vi "Main.vi"() -> ()   [LabVIEW 2017, in "Client.lvlib"]
uses:
  Client.lvlib
  CommsFrameWork.lvlib
  CommsServer.lvlib
  LabVIEWHTTPClient.lvlib
  ClientErrorHandler.lvlib
  ClientLogger.lvlib
  UI_API.lvlib
panel:
  out "Prio 4":u32(colorbox)
  out "Prio 3":u32(colorbox)
  out "Prio 2":u32(colorbox)
  out "Prio 1":u32(colorbox)
  in  "Filter Preset":T1(ring)
  out "Time to Refresh":dbl(slide) scale=0.0..10.0
  out "Connection Quality":dbl(knob) scale=0.0..10.0
  out "Connected?":bool
  out "Last Update":timestamp
  in  "Refresh":bool
  in  "AE Level":enum16{"AE / ELP", "AE Intern"}(ring)
  in  "AE Groups":i32[](listbox)
  in  "SRs Tab":enum32{"Unassigned", "Assigned", "Debug"}(tab)
  out "Unassigned Sorted SRs":string[][](table)
  out "Assigned Sorted SRs":string[][](table)
  out "INI Content":string
  out "INI Path":path
  in  "Read INI":bool
  out "Last Error Detected":errorcluster
  in  "Text":string="Manual Log Entry"
  in  "Type":string="Event"
  in  "Generate Log Entry":bool
  in  "Injected Error":errorcluster
  in  "Generate Error":bool
  # "Priority 1"
  # "Priority 3"
  # "Priority 2"
  # "Priority 4"
  # "Manual Controls"
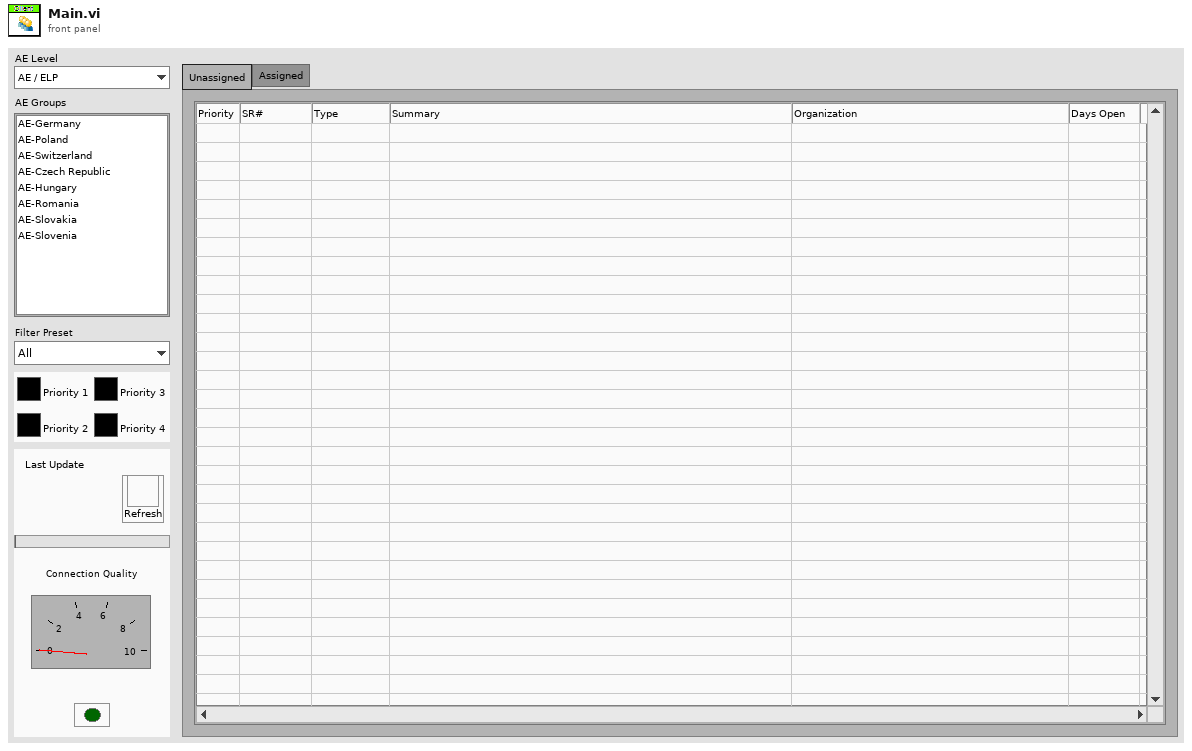
[diagram p1: front panel]
types:
  T1 = enum16{"All", "Eastern Europe", "DACH", "Custom"}
  T2 = cluster{"ErrorEventReg":refnum<event-registration>, "ErrorEvent":refnum<user-event>, "Queues":cluster{"MHLClient":refnum<queue>, "ErrorHandler":refnum<queue>, "EventHandler":refnum<queue>, "ConnectionHandler":refnum<queue>, "UIHandler":refnum<queue>, "Logger":refnum<queue>}}
  T3 = typedef "LVPoint32TypeDef.ctl" = cluster{"Horizontal":i32, "Vertical":i32}
  T4 = cluster{"Assigned SRs":refnum<vi>, "Unassigned SRs":refnum<vi>, "AE Level":refnum<vi>, "AE Groups":refnum<vi>}
  T5 = cluster{"SR Number":i64, "AE Group":enum32{"NaN", "AE-Germany", "AE-Poland", "AE-Switzerland", "AE-Czech Republic", "AE-Hungary", "AE-Romania", "AE-Slovakia", "AE-Slovenia"}, "SR Owner":string, "Summary":string, "SR Status":enum32{"NaN", "Caller Abandoned", "Created in Error", "Declined to Purchase Support", "Expired", "Forum Resolved AE", "Forum Resolved Customer", "IN WORK", "IN WORK Collab with AES", "IN WORK Collab with PSE", "IN WORK Collab with SE", "IN WORK Escalation", "IN WORK Customer Added Note", "Open", "Potentially Resolved", "POC Resolved", "Resolved", "RMA Waiting on Customer", "RMA Open", "RMA In Progress", "RMA Closed - DOA", "RMA Closed", "RMA Approved for Return", "Project Complete", "Presumed Resolved", "IN WORK Wait on Customer"}, "Days Open":dbl, "Prio":enum16{"Prio 1", "Prio 2", "Prio 3", "Prio 4"}, "SR Type":enum32{"NaN", "ATE Core Configurations (BYOATE)", "Activation", "BioBench", "CAN", "CM C Series", "Calibration", "Consulting Services", "CounterTimer", "DAQExpress", "DASYLab", "DIAdem", "DMM", "DSA HW", "Digital_IO", "FIRST (NIC Only)", "FieldBus", "FieldPoint", "Functional Savety", "GATI", "GPIB", "HMI and Industrial PCs", "HiQ", "HighSpeedDigital_IO", "IMAQ", "IOTech Vibration", "Industrial Communications", "InsightCM", "LV", "LV CD&Sim", "LV Comms", "LV Controls Add-Ons", "LV Embedded", "LV MathScript RT", "LV NXG", "LV NXT", "LVDSC", "LVFPGA", "LVPDA and LV Touch Panel", "LVRT", "LabWindows_CVI", "Lookout", "MATRIXx", "MStudioDotNet", "MStudioVisualBasic", "MStudioVisualC", "Measure (Legacy)", "Motion", "MultifunctionDAQ", "Multimedia Test HW/SW", "Multisim (EWB)", "NI Update Service", "OPC Servers", "Optical (OSI)", "PXI Controllers, Chassis, MXI", "PXI Timing and Sync", "Power Supplies and SMUs", "Powertrain Controls", "RAID", "RF", "RF Software", "RIO", "SC Express", "SCC", "SCXI", "SPEEDY-33 (Hyperception)", "STS", "ScopeDigitizers", "Serial", "Signal Sources", "SignalCondOther", "SignalExpress", "Software Defined Intruments", "Sound and Vibration SW", "Switch Executive", "Switches", "TestStand", "USRP", "Ultiboard (EWB)", "VBench", "VI Logger", "VXI_MXI", "VeriStand", "VisionSW", "VolumeLicenseMgr", "WSN", "Web UI Builder", "myRIO"}, "Service Level":string, "Last Updated":timestamp, "First Name":string, "Last Name":string, "Organisation Name":string, "Creation Date":timestamp, "Needs Merging?":bool, "English Flag?":bool}[]
  T6 = cluster{"Connection Quality":dbl, "Last Update":timestamp}
  T7 = enum16{"SR Number", "AE Group", "SR Owner", "Summary", "SR Status", "Days Open", "Prio", "SR Type", "Service Level", "Last Updated", "First Name", "Last Name", "Organisation Name", "Creation Date", "Needs Merging?", "English Flag?"}[]
  T8 = cluster{"Connection Data":cluster{"IP":string, "Port":string, "ClientName":string}}
  T9 = cluster{"SR#":dbl, "Group":string, "Owner":string, "Problem Summary":string, "Last Updated":timestamp, "Customer First Name":string, "Customer Last Name":string, "Company":string, "Created On":timestamp, "SR Type":string, "Status":string, "Service Level":string, "Channel":string, "Days Open":dbl}[]
  T10 = cluster{"IP":string, "Port":string, "ClientName":string}
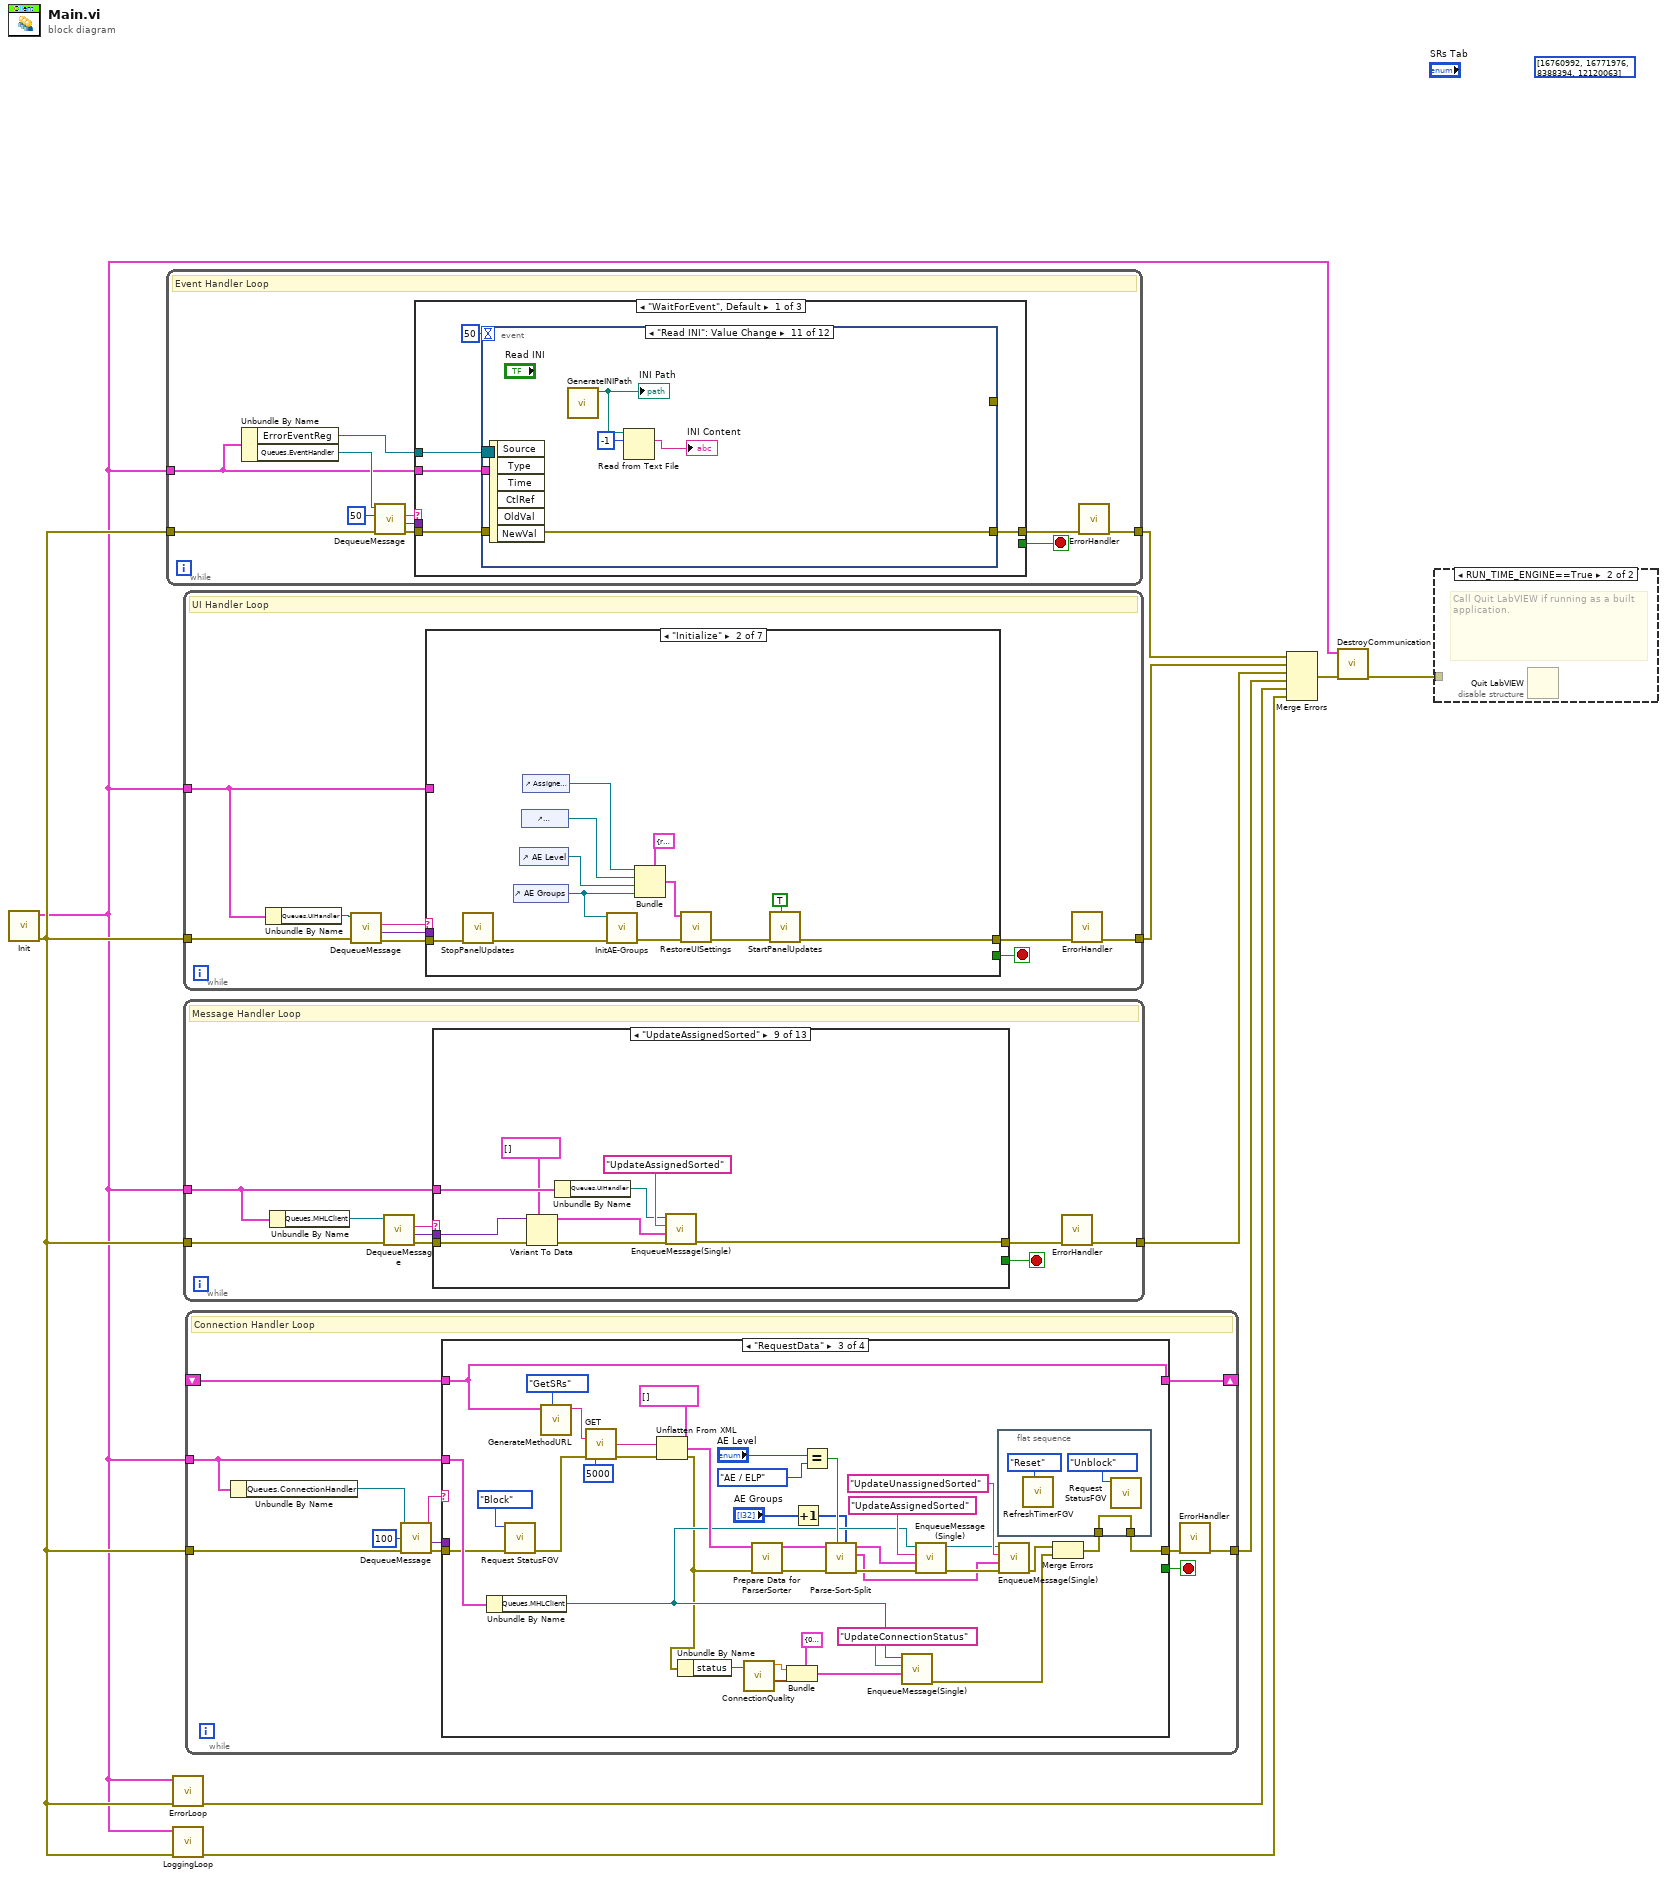
[diagram p0: block diagram]
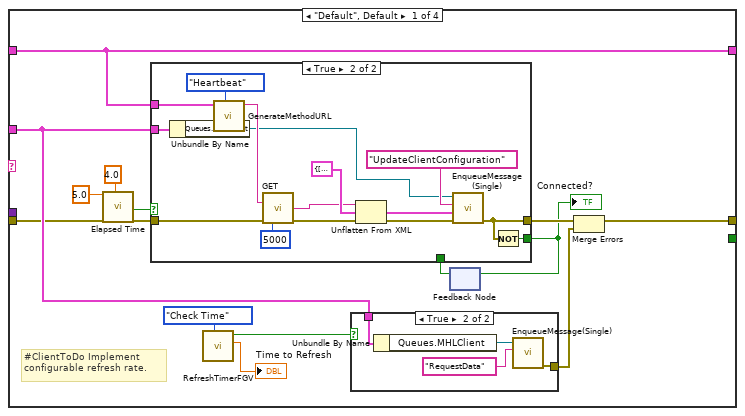
[diagram p2: hidden frame]
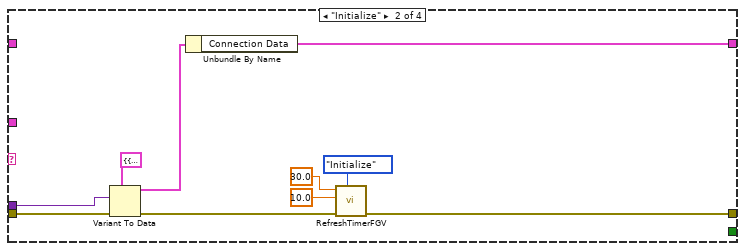
[diagram p5: hidden frame]
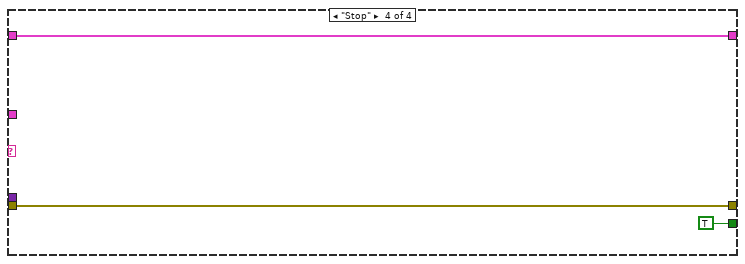
[diagram p6: hidden frame]
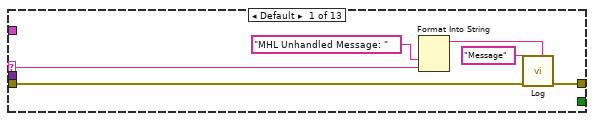
[diagram p7: hidden frame]
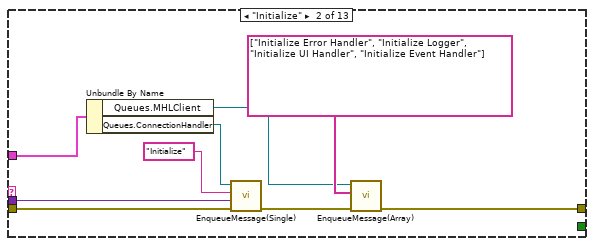
[diagram p8: hidden frame]
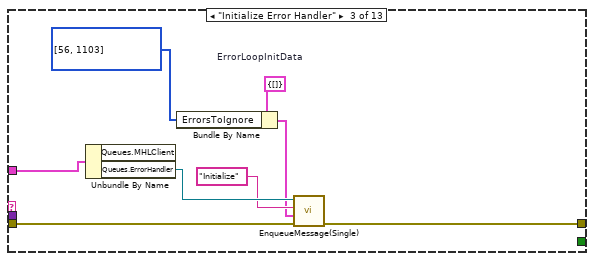
[diagram p9: hidden frame]
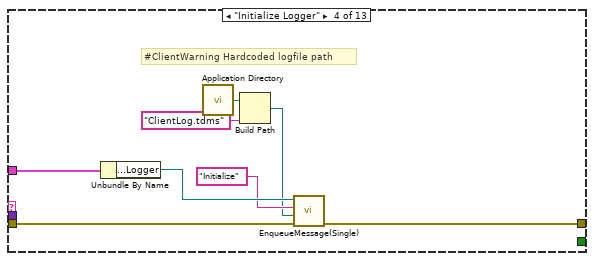
[diagram p10: hidden frame]
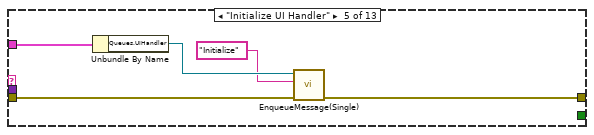
[diagram p11: hidden frame]
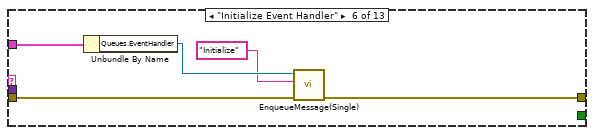
[diagram p12: hidden frame]
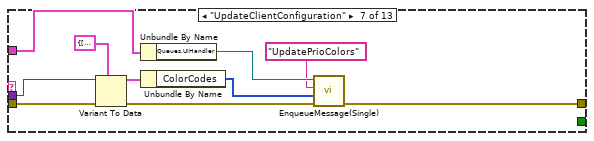
[diagram p13: hidden frame]
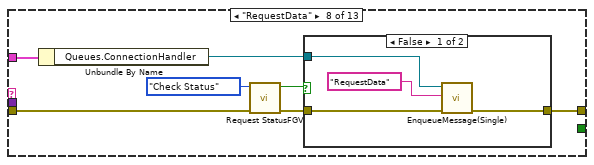
[diagram p14: hidden frame]
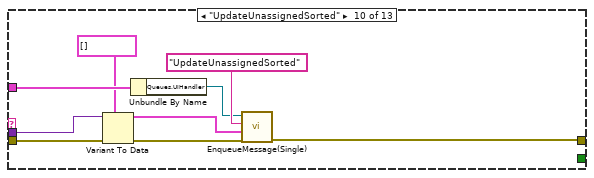
[diagram p16: hidden frame]
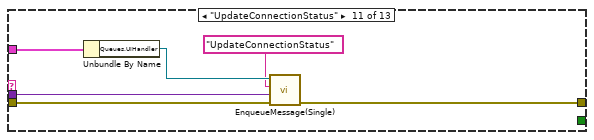
[diagram p17: hidden frame]
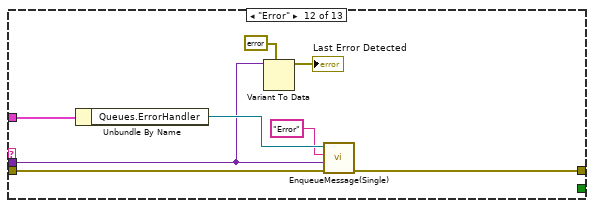
[diagram p18: hidden frame]
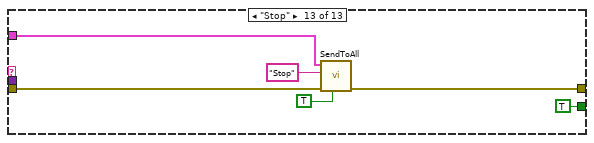
[diagram p19: hidden frame]
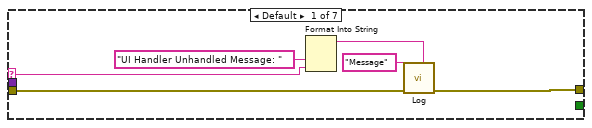
[diagram p20: hidden frame]
diagram:
  (unwired) u32[] [16760992, 16771976, 8388394, 12120063] ("Array")
  n1 = call "Init.vi"() -> ("Error Out"=w4:errorcluster, "Message Queues"=w3:T2)  [unwired: 10 in]
  n2 = while {
    tunnel: w3 -> [w13]
    tunnel: w4 -> [w20]
    tunnel: [w14] -> w9
    stop <- w16 stop-if-true
    # "Event Handler Loop"
    n3 = Unbundle By Name(w13) -> ("ErrorEventReg"=w12:refnum<event-registration>, "Queues.EventHandler"=w21:refnum<queue>)
    n4 = call "DequeueMessage.vi"("error in (no error)"=w20, "timeout ms (-1)"=50, "Message Queue"=w21) -> ("error out"=w18:errorcluster, "Message Data"=w17:variant, "Message"=w19:string)  [unwired: 4 in, 2 out]
    n5 = case shown="\"WaitForEvent\", Default" w19 {
      tunnel: w18 -> [w26 w144 w147]
      tunnel: [w23 w143 w147] -> w15
      tunnel: w17 -> [_ _ _]
      tunnel: [_ _ TRUE] -> w16
      tunnel: w13 -> [w25 w142 _]
      tunnel: w12 -> [w22 _ _]
      frame "WaitForEvent", Default {
        n6 = event shown="[10] \"Read INI\": Value Change" {
          selector: w22 -> [_ _ _ _ _ _ _ _ _ _ _ _]
          dyn-events: _ -> [_ _ _ _ _ _ _ _ _ _ _ _]
          timeout: 50 -> [_ _ _ _ _ _ _ _ _ _ _ _]
          tunnel: w26 -> [w29 w35 w48 w60 w62 w69 w73 w81 w98 w110 w125 w127]
          tunnel: w25 -> [w31 w37 w56 _ _ w68 w75 _ w101 _ _ _]
          tunnel: [w30 w33 w49 w60 w61 w65 w72 w80 w99 w109 w125 w126] -> w23
          tunnel: [_ _ _ _ _ _ w70 _ _ _ _ _] -> _
          event Timeout {
            n7 = event-data() -> ()  [unwired: 1 in, 3 out]
            n8 = Unbundle By Name(w31) -> ("Queues.EventHandler"=w27:refnum<queue>)
            n9 = call "EnqueueMessage(Single).vi"("error in (no error)"=w29, "Message"="WaitForEvent", "Message Queue"=w27) -> ("error out"=w30:errorcluster)  [unwired: 7 in, 1 out]
          }
          event "Filter Preset": Value Change {
            # "#ClientToDo Replace hardwired values with configuration data."
            n10 = event-data() -> ("NewVal"=w38:T1)  [unwired: 1 in]
            n11 = case shown="\"Eastern Europe\"" w38 {
              tunnel: w35 -> [w39 w41 w43 w45]
              tunnel: [w39 w41 w43 w45] -> w34
              frame "All", Default {
                n12 = property on="AE Groups" class="LstBox (strict)"("Value"=i32[] [0, 1, 2, 3, 4, 5, 6, 7] ("Value (Signaling)")) -> ()  [unwired: 2 in, 2 out]
              }
              frame "Eastern Europe" {
                n13 = property on="AE Groups" class="LstBox (strict)"("Value"=i32[] [1, 3, 4, 5, 6, 7] ("Value (Signaling)")) -> ()  [unwired: 2 in, 2 out]
              }
              frame "DACH" {
                n14 = property on="AE Groups" class="LstBox (strict)"("Value"=i32[] [0, 2] ("Value (Signaling)")) -> ()  [unwired: 2 in, 2 out]
              }
              frame "Custom" {
              }
            }
            n15 = Unbundle By Name(w37) -> ("Queues.MHLClient"=w36:refnum<queue>)
            n16 = call "EnqueueMessage(Single).vi"("error in (no error)"=w34, "Message"="RequestData", "Message Queue"=w36) -> ("error out"=w33:errorcluster)  [unwired: 7 in, 1 out]
          }
          event "AE Level", "AE Groups": Value Change {
            n17 = event-data() -> ("CtlRef"=w54:refnum<vi>)  [unwired: 1 in]
            n18 = call "StopPanelUpdates.vi"("Error In"=w48) -> ("Error Out"=w47:errorcluster)  [unwired: 10 in]
            n19 = property class="Ctl"(reference=w54) -> ("Label.Text"=w53:string)  [unwired: 1 in, 2 out]
            n20 = Unbundle By Name(w56) -> ("Queues.MHLClient"=w57:refnum<queue>)
            n21 = case shown="\"AE Groups\"" w53 {
              frame "False", Default {
              }
              frame "AE Groups" {
                n22 = local write "Filter Preset"(T1."Custom" ("Filter Preset")) -> ()
              }
            }
            n23 = call "EnqueueMessage(Single).vi"("error in (no error)"=w47, "Message"="RequestData", "Message Queue"=w57) -> ("error out"=w46:errorcluster)  [unwired: 7 in, 1 out]
            n24 = control-ref of="Unassigned Sorted SRs"() -> (w52:refnum<vi>)
            n25 = control-ref of="Assigned Sorted SRs"() -> (w51:refnum<vi>)
            n26 = Build Array(w52, w51) -> (w50:refnum<vi>[])
            n27 = call "ResetTablesToTopPosition.vi"("Error In"=w46, "Table Refnum Array"=w50) -> ("Error Out"=w49:errorcluster)  [unwired: 9 in]
          }
          event "Generate Error": Value Change {
            # "#ClientWarning Debug Feature"
            n28 = event-data() -> ()  [unwired: 1 in, 6 out]
            n29 = call "ErrorHandler.vi"("error in (no error)"="Injected Error") -> ()  [unwired: 10 in, 1 out]
          }
          event "Generate Log Entry": Value Change {
            # "#ClientWarning Debug Feature"
            n30 = event-data() -> ()  [unwired: 1 in, 6 out]
            n31 = call "Log.vi"("LogMessage"="Text", "Type"="Type", "Error In"=w62) -> ("Error Out"=w61:errorcluster)  [unwired: 8 in]
          }
          event "Refresh": Value Change {
            n32 = event-data() -> ()  [unwired: 1 in, 1 out]
            n33 = Unbundle By Name(w68) -> ("Queues.MHLClient"=w67:refnum<queue>)
            n34 = call "EnqueueMessage(Single).vi"("error in (no error)"=w69, "Message"="RequestData", "Message Queue"=w67) -> ("error out"=w65:errorcluster)  [unwired: 7 in, 1 out]
          }
          event User Event {
            n35 = event-data() -> ("status"=w78:bool, "code"=w77:i32, "source"=w76:string)  [unwired: 1 in]
            n36 = Unbundle By Name(w75) -> ("Queues.MHLClient"=w74:refnum<queue>)
            n37 = Bundle(cluster=errorcluster {"status"=FALSE, "code"=0, "source"=""} ("error constant"), "status"=w78, "code"=w77, "source"=w76) -> (w70:errorcluster)
            n38 = call "EnqueueMessage(Single).vi"("error in (no error)"=w73, "Message"="Stop", "Message Queue"=w74) -> ("error out"=w72:errorcluster)  [unwired: 7 in, 1 out]
          }
          event "Unassigned Sorted SRs": Shortcut Menu Selection (User) {
            # "#ClientToDo Adapt SR# finding to configurable columns"
            n39 = event-data() -> ("ItemTag"=w82:string, "CtlRef"=w84:refnum<vi>, "Coords"=w83:T3)  [unwired: 1 in]
            n40 = case shown="\"Copy SR#\", Default" w82 {
              tunnel: w84 -> [w90 w95]
              tunnel: w83 -> [w89 w93]
              tunnel: [w85 w92] -> w80
              tunnel: w81 -> [w86 w91]
              frame "Open Screenpop" {
                # "#ClientToDo URL from config data."
                n41 = call "Open Screenpop.vi"("Screenpop URL Prefix"="http://force.natinst.com:8000/pls/ebiz/niae_screenpop.main?p_incident_number=", "SR# Cloumn Header"="SR#" ("SR Cloumn Header"), "Error In"=w86, "Coordinates"=w89, "Table Reference"=w90) -> ("Error Out"=w85:errorcluster)  [unwired: 6 in]
              }
              frame "Copy SR#", Default {
                n42 = call "Copy SR Num to Clipboard.vi"("SR Cloumn Header"="SR#", "Error In"=w91, "Coordinates"=w93, "Table Reference"=w95) -> ("Error Out"=w92:errorcluster)  [unwired: 7 in]
              }
            }
          }
          event Panel Close? {
            n43 = event-data() -> ()  [unwired: 1 in, 1 out]
            n44 = Unbundle By Name(w101) -> ("Queues.MHLClient"=w100:refnum<queue>)
            n45 = call "QuitDialog.vi"("Error In"=w98) -> ("Error Out"=w97:errorcluster, "OK Clicked?"=w96:bool)  [unwired: 9 in]
            n46 = case shown="True" w96 {
              tunnel: w100 -> [_ w108]
              tunnel: [w103 w107] -> w99
              tunnel: w97 -> [w103 w106]
              frame False {
              }
              frame True {
                n47 = call "EnqueueMessage(Single).vi"("Priority Message? (F)"=TRUE, "error in (no error)"=w106, "Message"="Stop", "Message Queue"=w108) -> ("error out"=w107:errorcluster)  [unwired: 6 in, 1 out]
              }
            }
            n48 = event-data("Discard?"=TRUE) -> ()  [unwired: 1 in, 1 out]
          }
          event Key Down? {
            # "#ClientWarning Debug Feature"
            n49 = event-data() -> ("ScanCode"=w115:i16, "PlatMods.Ctrl"=w113:bool, "PlatMods.Shift"=w112:bool)  [unwired: 1 in]
            n50 = Equal?(x=i16 32 ("ScanCode"), y=w115) -> (x = y?=w114:bool)
            n51 = Compound Arithmetic op=AND(w114, w113, w112) -> (w111:bool)
            n52 = case shown="True" w111 {
              tunnel: w110 -> [w117 w121]
              tunnel: [w117 w120] -> w109
              frame False {
              }
              frame True {
                n53 = control-ref of="SRs Tab"() -> (w119:refnum<vi>)
                n54 = call "ToggleTab.vi"("Error In"=w121, "Tab Index"=2, "TabCtl Refnum"=w119) -> ("Error Out"=w120:errorcluster)  [unwired: 8 in]
              }
            }
            n55 = event-data() -> ()  [unwired: 2 in, 1 out]
          }
          event "Read INI": Value Change {
            n56 = event-data() -> ()  [unwired: 1 in, 6 out]
            n57 = call "GenerateINIPath.vi"() -> ("INI Path"=w124:path)  [unwired: 11 in]
            "INI Path" <- w124
            n58 = Read from Text File(file (use dialog)=w124, count=-1) -> (text=→"INI Content":string)  [unwired: 2 in, 3 out]
          }
          event "Assigned Sorted SRs": Shortcut Menu Selection (User) {
            # "#ClientToDo Adapt SR# finding to configurable columns"
            n59 = event-data() -> ("ItemTag"=w130:string, "CtlRef"=w129:refnum<vi>, "Coords"=w128:T3)  [unwired: 1 in]
            n60 = case shown="\"Open Screenpop\"" w130 {
              tunnel: w129 -> [w136 w141]
              tunnel: w128 -> [w135 w139]
              tunnel: w127 -> [w132 w138]
              tunnel: [w131 w137] -> w126
              frame "Open Screenpop" {
                # "#ClientToDo URL from config data."
                n61 = call "Open Screenpop.vi"("Screenpop URL Prefix"="http://force.natinst.com:8000/pls/ebiz/niae_screenpop.main?p_incident_number=", "SR# Cloumn Header"="SR#" ("SR Cloumn Header"), "Error In"=w132, "Coordinates"=w135, "Table Reference"=w136) -> ("Error Out"=w131:errorcluster)  [unwired: 6 in]
              }
              frame "Copy SR#", Default {
                n62 = call "Copy SR Num to Clipboard.vi"("SR Cloumn Header"="SR#", "Error In"=w138, "Coordinates"=w139, "Table Reference"=w141) -> ("Error Out"=w137:errorcluster)  [unwired: 7 in]
              }
            }
          }
        }
      }
      frame "Initialize" {
        n63 = Unbundle By Name(w142) -> ("Queues.EventHandler"=w146:refnum<queue>)
        n64 = call "EnqueueMessage(Single).vi"("error in (no error)"=w144, "Message"="WaitForEvent", "Message Queue"=w146) -> ("error out"=w143:errorcluster)  [unwired: 7 in, 1 out]
      }
      frame "Stop" {
      }
    }
    n65 = call "ErrorHandler.vi"("error in (no error)"=w15) -> ("error out"=w14:errorcluster)  [unwired: 10 in]
  }
  n66 = call "ErrorLoop.vi"("Error In"=w4, "Message Queues"=w3) -> ("Error Out"=w5:errorcluster)  [unwired: 9 in]
  n67 = call "LoggingLoop.vi"("Error In"=w4, "Communication References"=w3) -> ("Error Out"=w2:errorcluster)  [unwired: 9 in]
  n68 = while {
    tunnel: w3 -> [w151]
    tunnel: w4 -> [w156]
    tunnel: [w149] -> w8
    stop <- w152 stop-if-true
    # "UI Handler Loop"
    n69 = Unbundle By Name(w151) -> ("Queues.UIHandler"=w157:refnum<queue>)
    n70 = call "DequeueMessage.vi"("error in (no error)"=w156, "Message Queue"=w157) -> ("error out"=w155:errorcluster, "Message Data"=w153:variant, "Message"=w154:string)  [unwired: 5 in, 2 out]
    n71 = case shown="\"Initialize\"" w154 {
      selector: w154 -> [w160 _ _ _ _ _ _]
      tunnel: w155 -> [w159 w168 w192 w208 w218 w229 w238]
      tunnel: [w158 w164 w176 w195 w217 w219 w237] -> w150
      tunnel: w153 -> [_ _ w193 w209 w216 w228 _]
      tunnel: [_ _ _ _ _ _ TRUE] -> w152
      tunnel: w151 -> [_ _ _ _ _ w221 _]
      frame Default {
        n72 = Format Into String("UI Handler Unhandled Message: " ("Type"), w160) -> (resulting string=w163:string)  [unwired: 3 in, 1 out]
        n73 = call "Log.vi"("LogMessage"=w163, "Type"="Message", "Error In"=w159) -> ("Error Out"=w158:errorcluster)  [unwired: 8 in]
      }
      frame "Initialize" {
        n74 = call "StopPanelUpdates.vi"("Error In"=w168) -> ("Error Out"=w167:errorcluster)  [unwired: 10 in]
        n75 = control-ref of="AE Groups"() -> (w171:refnum<vi>)
        n76 = control-ref of="AE Level"() -> (w173:refnum<vi>)
        n77 = control-ref of="Unassigned Sorted SRs"() -> (w174:refnum<vi>)
        n78 = control-ref of="Assigned Sorted SRs"() -> (w175:refnum<vi>)
        n79 = call "InitAE-Groups.vi"("Error In"=w167, "LstBox Refnum"=w171) -> ("Error Out"=w170:errorcluster)  [unwired: 9 in]
        n80 = Bundle(cluster=T4 {"Assigned SRs"=refnum, "Unassigned SRs"=refnum, "AE Level"=refnum, "AE Groups"=refnum} ("UI References"), "Assigned SRs"=w175, "Unassigned SRs"=w174, "AE Level"=w173, "AE Groups"=w171) -> (w169:T4)
        n81 = call "RestoreUISettings.vi"("Error In"=w170, "UI References"=w169) -> ("Error Out"=w166:errorcluster)  [unwired: 9 in]
        n82 = call "StartPanelUpdates.vi"("Ignore Error In"=TRUE, "Error In"=w166) -> ("Error Out"=w164:errorcluster)  [unwired: 9 in]
      }
      frame "UpdateAssignedSorted" {
        w190 = T7 [enum."SR Owner", enum."SR Number", enum."Summary", enum."Organisation Name"] items=["SR Number", "AE Group", "SR Owner", "Summary", "SR Status", "Days Open", "Prio", "SR Type", "Service Level", "Last Updated", "First Name", "Last Name", "Organisation Name", "Creation Date", "Needs Merging?", "English Flag?"] ("Fields to include")
        # "#ClientToDo Implement configurable columns."
        n83 = Variant To Data(error in=w192, type=T5 [] ("SR List In"), Variant=w193) -> (data=w187:T5, error out=w180:errorcluster)
        n84 = call "StopPanelUpdates.vi"("Error In"=w180) -> ("Error Out"=w179:errorcluster)  [unwired: 10 in]
        n85 = call "SRListToTable.vi"("Fields to include"=w190, "Error In"=w179, "SR List In"=w187) -> ("Error Out"=w188:errorcluster, "2D String Array for Table"=→"Assigned Sorted SRs":string[][])  [unwired: 7 in]
        n86 = local read "Prio 1"() -> (w185:u32)
        n87 = local read "Prio 2"() -> (w184:u32)
        n88 = local read "Prio 3"() -> (w183:u32)
        n89 = local read "Prio 4"() -> (w182:u32)
        n90 = control-ref of="Assigned Sorted SRs"() -> (w186:refnum<vi>)
        n91 = Build Array(w185, w184, w183, w182) -> (w181:u32[])
        n92 = call "PriorityColoring.vi"("Color Array"=w181, "Error In"=w188, "Tbl Refnum"=w186, "SR List In"=w187) -> ("Error Out"=w178:errorcluster)  [unwired: 7 in]
        n93 = call "StartPanelUpdates.vi"("Ignore Error In"=TRUE, "Error In"=w178) -> ("Error Out"=w176:errorcluster)  [unwired: 9 in]
      }
      frame "UpdateUnassignedSorted" {
        w210 = T7 [enum."Prio", enum."SR Number", enum."SR Type", enum."Summary", enum."Organisation Name", enum."Days Open", enum."First Name", enum."Last Name"] items=["SR Number", "AE Group", "SR Owner", "Summary", "SR Status", "Days Open", "Prio", "SR Type", "Service Level", "Last Updated", "First Name", "Last Name", "Organisation Name", "Creation Date", "Needs Merging?", "English Flag?"] ("Fields to include")
        # "#ClientToDo Implement configurable columns."
        n94 = Variant To Data(error in=w208, type=T5 [] ("SR List In"), Variant=w209) -> (data=w205:T5, error out=w198:errorcluster)
        n95 = call "StopPanelUpdates.vi"("Error In"=w198) -> ("Error Out"=w197:errorcluster)  [unwired: 10 in]
        n96 = call "SRListToTable.vi"("Fields to include"=w210, "Error In"=w197, "SR List In"=w205) -> ("Error Out"=w206:errorcluster, "2D String Array for Table"=→"Unassigned Sorted SRs":string[][])  [unwired: 7 in]
        n97 = local read "Prio 1"() -> (w203:u32)
        n98 = local read "Prio 2"() -> (w202:u32)
        n99 = local read "Prio 3"() -> (w201:u32)
        n100 = local read "Prio 4"() -> (w200:u32)
        n101 = control-ref of="Unassigned Sorted SRs"() -> (w204:refnum<vi>)
        n102 = Build Array(w203, w202, w201, w200) -> (w199:u32[])
        n103 = call "PriorityColoring.vi"("Color Array"=w199, "Error In"=w206, "Tbl Refnum"=w204, "SR List In"=w205) -> ("Error Out"=w196:errorcluster)  [unwired: 7 in]
        n104 = call "StartPanelUpdates.vi"("Ignore Error In"=TRUE, "Error In"=w196) -> ("Error Out"=w195:errorcluster)  [unwired: 9 in]
      }
      frame "UpdateConnectionStatus" {
        n105 = Variant To Data(error in=w218, type=T6 {"Connection Quality"=0.0, "Last Update"=timestamp(0 s since 1904-01-01)} ("Connection Status"), Variant=w216) -> (data=w214:T6, error out=w217:errorcluster)
        n106 = Unbundle(w214) -> ("Connection Quality"=→"Connection Quality":dbl, "Last Update"=→"Last Update":timestamp)
      }
      frame "UpdatePrioColors" {
        # "#ClientToDo Replace hacky first update when centralized timing becomes available."
        n107 = Variant To Data(error in=w229, type=u32[] [] ("ColorCodes"), Variant=w228) -> (data=w227:u32[], error out=w220:errorcluster)
        n108 = Index Array(array=w227) -> (element #1=→"Prio 1":u32, element #2=→"Prio 2":u32, element #3=→"Prio 3":u32, element #4=→"Prio 4":u32)  [unwired: 4 in]
        n109 = First Call?() -> (First Call?: T/F=w222:bool)
        n110 = case shown="True" w222 {
          tunnel: w221 -> [_ w235]
          tunnel: w220 -> [w231 w233]
          tunnel: [w231 w232] -> w219
          frame False {
          }
          frame True {
            n111 = Unbundle By Name(w235) -> ("Queues.MHLClient"=w234:refnum<queue>)
            n112 = call "EnqueueMessage(Single).vi"("error in (no error)"=w233, "Message"="RequestData", "Message Queue"=w234) -> ("error out"=w232:errorcluster)  [unwired: 7 in, 1 out]
          }
        }
      }
      frame "Stop" {
        n113 = control-ref of="AE Groups"() -> (w241:refnum<vi>)
        n114 = control-ref of="AE Level"() -> (w242:refnum<vi>)
        n115 = control-ref of="Unassigned Sorted SRs"() -> (w243:refnum<vi>)
        n116 = control-ref of="Assigned Sorted SRs"() -> (w244:refnum<vi>)
        n117 = Bundle(cluster=T4 {"Assigned SRs"=refnum, "Unassigned SRs"=refnum, "AE Level"=refnum, "AE Groups"=refnum} ("UI References"), "Assigned SRs"=w244, "Unassigned SRs"=w243, "AE Level"=w242, "AE Groups"=w241) -> (w239:T4)
        n118 = call "SaveUISettings.vi"("Error In"=w238, "UI References"=w239) -> ("Error Out"=w237:errorcluster)  [unwired: 9 in]
      }
    }
    n119 = call "ErrorHandler.vi"("error in (no error)"=w150) -> ("error out"=w149:errorcluster)  [unwired: 10 in]
  }
  n120 = while {
    tunnel: w3 -> [w248]
    tunnel: w4 -> [w254]
    tunnel: [w246] -> w7
    stop <- w249 stop-if-true
    # "Message Handler Loop"
    n121 = Unbundle By Name(w248) -> ("Queues.MHLClient"=w253:refnum<queue>)
    n122 = call "DequeueMessage.vi"("error in (no error)"=w254, "Message Queue"=w253) -> ("error out"=w250:errorcluster, "Message Data"=w251:variant, "Message"=w252:string)  [unwired: 5 in, 2 out]
    n123 = case shown="\"UpdateAssignedSorted\"" w252 {
      selector: w252 -> [w259 _ _ _ _ _ _ _ _ _ _ _ _]
      tunnel: w251 -> [_ w269 _ _ _ _ w304 _ w324 w333 w339 w344 _]
      tunnel: w250 -> [w256 w266 w276 w284 w289 w294 w305 w308 w323 w332 w341 w346 w353]
      tunnel: [w255 w262 w273 w281 w286 w291 w300 w312 w318 w327 w340 w345 w352] -> w247
      tunnel: [_ _ _ _ _ _ _ _ _ _ _ _ TRUE] -> w249
      tunnel: w248 -> [_ w268 w277 w285 w290 w295 w298 w311 w326 w335 w338 w349 w351]
      frame Default {
        n124 = Format Into String("MHL Unhandled Message: " ("Type"), w259) -> (resulting string=w257:string)  [unwired: 3 in, 1 out]
        n125 = call "Log.vi"("LogMessage"=w257, "Type"="Message", "Error In"=w256) -> ("Error Out"=w255:errorcluster)  [unwired: 8 in]
      }
      frame "Initialize" {
        n126 = Unbundle By Name(w268) -> ("Queues.MHLClient"=w261:refnum<queue>, "Queues.ConnectionHandler"=w267:refnum<queue>)
        n127 = call "EnqueueMessage(Single).vi"("error in (no error)"=w266, "Message Data"=w269, "Message"="Initialize", "Message Queue"=w267) -> ("error out"=w264:errorcluster)  [unwired: 6 in, 1 out]
        n128 = call "EnqueueMessage(Array).vi"("error in (no error)"=w264, "Message Array"=string[] ["Initialize Error Handler", "Initialize Logger", "Initialize UI Handler", "Initialize Event Handler"], "Message Queue"=w261) -> ("error out"=w262:errorcluster)  [unwired: 7 in, 1 out]
      }
      frame "Initialize Error Handler" {
        w272 = cluster{"ErrorsToIgnore":i32[]} {"ErrorsToIgnore"=[]}  # ErrorLoopInitData
        n129 = Unbundle By Name(w277) -> ("Queues.ErrorHandler"=w275:refnum<queue>)  [unwired: 1 out]
        n130 = Bundle By Name(cluster=w272, "ErrorsToIgnore"=i32[] [56, 1103]) -> (w271:cluster{"ErrorsToIgnore":i32[]})
        n131 = call "EnqueueMessage(Single).vi"("error in (no error)"=w276, "Message Data"=w271, "Message"="Initialize", "Message Queue"=w275) -> ("error out"=w273:errorcluster)  [unwired: 6 in, 1 out]
      }
      frame "Initialize Logger" {
        # "#ClientWarning Hardcoded logfile path"
        n132 = Unbundle By Name(w285) -> ("Queues.Logger"=w283:refnum<queue>)
        n133 = call "Application Directory.vi"() -> ("Application Directory"=w280:path)
        n134 = Build Path(base path=w280, name or relative path="ClientLog.tdms") -> (appended path=w278:path)
        n135 = call "EnqueueMessage(Single).vi"("error in (no error)"=w284, "Message Data"=w278, "Message"="Initialize", "Message Queue"=w283) -> ("error out"=w281:errorcluster)  [unwired: 6 in, 1 out]
      }
      frame "Initialize UI Handler" {
        n136 = Unbundle By Name(w290) -> ("Queues.UIHandler"=w288:refnum<queue>)
        n137 = call "EnqueueMessage(Single).vi"("error in (no error)"=w289, "Message"="Initialize", "Message Queue"=w288) -> ("error out"=w286:errorcluster)  [unwired: 7 in, 1 out]
      }
      frame "Initialize Event Handler" {
        n138 = Unbundle By Name(w295) -> ("Queues.EventHandler"=w293:refnum<queue>)
        n139 = call "EnqueueMessage(Single).vi"("error in (no error)"=w294, "Message"="Initialize", "Message Queue"=w293) -> ("error out"=w291:errorcluster)  [unwired: 7 in, 1 out]
      }
      frame "UpdateClientConfiguration" {
        n140 = Variant To Data(error in=w305, type=cluster{"ColorCodes":u32[]} {"ColorCodes"=[16711680, 6618880, 16774745, 9567230]} ("ClientConfig"), Variant=w304) -> (data=w302:cluster{"ColorCodes":u32[]}, error out=w301:errorcluster)
        n141 = Unbundle By Name(w298) -> ("Queues.UIHandler"=w297:refnum<queue>)
        n142 = Unbundle By Name(w302) -> ("ColorCodes"=w299:u32[])
        n143 = call "EnqueueMessage(Single).vi"("error in (no error)"=w301, "Message Data"=w299, "Message"="UpdatePrioColors", "Message Queue"=w297) -> ("error out"=w300:errorcluster)  [unwired: 6 in, 1 out]
      }
      frame "RequestData" {
        n144 = Unbundle By Name(w311) -> ("Queues.ConnectionHandler"=w310:refnum<queue>)
        n145 = call "Request StatusFGV.vi"("Error In"=w308, "Command"=enum16{"Block", "Unblock", "Check Status"}."Check Status") -> ("Error Out"=w307:errorcluster, "Blocked?"=w306:bool)  [unwired: 8 in]
        n146 = case shown="False" w306 {
          tunnel: [w316 w317] -> w312
          tunnel: w310 -> [w315 _]
          tunnel: w307 -> [w313 w317]
          frame False {
            n147 = call "EnqueueMessage(Single).vi"("error in (no error)"=w313, "Message"="RequestData", "Message Queue"=w315) -> ("error out"=w316:errorcluster)  [unwired: 7 in, 1 out]
          }
          frame True {
          }
        }
      }
      frame "UpdateAssignedSorted" {
        n148 = Variant To Data(error in=w323, type=T5 [] ("SR List In"), Variant=w324) -> (data=w320:T5, error out=w319:errorcluster)
        n149 = Unbundle By Name(w326) -> ("Queues.UIHandler"=w322:refnum<queue>)
        n150 = call "EnqueueMessage(Single).vi"("error in (no error)"=w319, "Message Data"=w320, "Message"="UpdateAssignedSorted", "Message Queue"=w322) -> ("error out"=w318:errorcluster)  [unwired: 6 in, 1 out]
      }
      frame "UpdateUnassignedSorted" {
        n151 = Variant To Data(error in=w332, type=T5 [] ("SR List In"), Variant=w333) -> (data=w329:T5, error out=w328:errorcluster)
        n152 = Unbundle By Name(w335) -> ("Queues.UIHandler"=w331:refnum<queue>)
        n153 = call "EnqueueMessage(Single).vi"("error in (no error)"=w328, "Message Data"=w329, "Message"="UpdateUnassignedSorted", "Message Queue"=w331) -> ("error out"=w327:errorcluster)  [unwired: 6 in, 1 out]
      }
      frame "UpdateConnectionStatus" {
        n154 = Unbundle By Name(w338) -> ("Queues.UIHandler"=w337:refnum<queue>)
        n155 = call "EnqueueMessage(Single).vi"("error in (no error)"=w341, "Message Data"=w339, "Message"="UpdateConnectionStatus", "Message Queue"=w337) -> ("error out"=w340:errorcluster)  [unwired: 6 in, 1 out]
      }
      frame "Error" {
        n156 = Unbundle By Name(w349) -> ("Queues.ErrorHandler"=w348:refnum<queue>)
        n157 = Variant To Data(type=errorcluster {"status"=FALSE, "code"=0, "source"=""} ("error constant"), Variant=w344) -> (data=→"Last Error Detected":errorcluster)  [unwired: 1 in, 1 out]
        n158 = call "EnqueueMessage(Single).vi"("error in (no error)"=w346, "Message Data"=w344, "Message"="Error", "Message Queue"=w348) -> ("error out"=w345:errorcluster)  [unwired: 6 in, 1 out]
      }
      frame "Stop" {
        n159 = call "SendToAll.vi"("Priority Message? (F)"=TRUE, "error in (no error)"=w353, "Message"="Stop", "Message Queues"=w351) -> ("error out"=w352:errorcluster)  [unwired: 7 in]
      }
    }
    n160 = call "ErrorHandler.vi"("error in (no error)"=w247) -> ("error out"=w246:errorcluster)  [unwired: 10 in]
  }
  n161 = while {
    tunnel: w3 -> [w361]
    shift-right: [w359] -> _
    shift-left: _ -> [w358]
    tunnel: w4 -> [w367]
    tunnel: [w356] -> w6
    stop <- w362 stop-if-true
    # "Connection Handler Loop"
    n162 = Unbundle By Name(w361) -> ("Queues.ConnectionHandler"=w366:refnum<queue>)
    n163 = call "DequeueMessage.vi"("error in (no error)"=w367, "timeout ms (-1)"=100, "Message Queue"=w366) -> ("error out"=w363:errorcluster, "Message Data"=w364:variant, "Message"=w365:string)  [unwired: 4 in, 2 out]
    n164 = case shown="\"RequestData\"" w365 {
      tunnel: w364 -> [_ w412 _ _]
      tunnel: w363 -> [w373 w413 w424 w456]
      tunnel: [w380 w407 w416 w456] -> w357
      tunnel: [_ _ _ TRUE] -> w362
      tunnel: w361 -> [w376 _ w446 _]
      tunnel: [w382 w409 w451 w455] -> w359
      tunnel: w358 -> [w382 _ w451 w455]
      frame "Default", Default {
        # "#ClientToDo Implement configurable refresh rate."
        n165 = call "Elapsed Time"("Time Target (s)"=5.0, "error in (no error)"=w373, "Set Start Time (s)"=4.0) -> ("Time has Elapsed"=w371:bool, "error out"=w372:errorcluster)  [unwired: 9 in, 6 out]
        n166 = call "RefreshTimerFGV.vi"("Command"=enum16{"Initialize", "Check Time", "Reset"}."Check Time") -> ("Time to Next Refresh"=→"Time to Refresh":dbl, "Refresh Now?"=w370:bool)  [unwired: 8 in, 1 out]
        n167 = case shown="True" w370 {
          tunnel: w376 -> [_ w403]
          tunnel: [_ w400] -> w381
          frame False {
          }
          frame True {
            n168 = Unbundle By Name(w403) -> ("Queues.MHLClient"=w402:refnum<queue>)
            n169 = call "EnqueueMessage(Single).vi"("Message"="RequestData", "Message Queue"=w402) -> ("error out"=w400:errorcluster)  [unwired: 8 in, 1 out]
          }
        }
        n170 = feedback #1() -> (w377:bool)  [unwired: 1 in]
        n171 = case shown="True" w371 {
          tunnel: w382 -> [_ w399]
          tunnel: w372 -> [w384 w397]
          tunnel: [w383 w395] -> w378
          tunnel: [w384 w394] -> w379
          tunnel: w377 -> [w383 _]
          tunnel: w376 -> [_ w392]
          frame False {
          }
          frame True {
            n172 = Unbundle By Name(w392) -> ("Queues.MHLClient"=w386:refnum<queue>)
            n173 = call "GenerateMethodURL.vi"("Method"=enum16{"Heartbeat", "GetSRs"}."Heartbeat", "TestClientData"=w399) -> ("String"=w396:string)  [unwired: 9 in]
            n174 = call "GET.vi"("url"=w396, "error in (no error)"=w397, "timeout (10000)"=5000) -> ("body"=w388:string, "error out"=w391:errorcluster)  [unwired: 9 in, 2 out]
            n175 = Unflatten From XML(xml string=w388, type=cluster{"ColorCodes":u32[]} {"ColorCodes"=[16711680, 6618880, 16774745, 9567230]} ("ClientConfig"), error in (no error)=w391) -> (value=w387:cluster{"ColorCodes":u32[]}, error out=w390:errorcluster)
            n176 = call "EnqueueMessage(Single).vi"("error in (no error)"=w390, "Message Data"=w387, "Message"="UpdateClientConfiguration", "Message Queue"=w386) -> ("error out"=w394:errorcluster)  [unwired: 6 in, 1 out]
            n177 = Not(x=w394) -> (.not. x?=w395:bool)
          }
        }
        "Connected?" <- w378
        n178 = feedback-in #1(w378) -> ()
        n179 = Merge Errors(w379, w381) -> (w380:errorcluster)
      }
      frame "Initialize" {
        n180 = Variant To Data(error in=w413, type=T8 {"Connection Data"={"IP"="", "Port"="", "ClientName"=""}} ("InternalData"), Variant=w412) -> (data=w410:T8, error out=w408:errorcluster)
        n181 = Unbundle By Name(w410) -> ("Connection Data"=w409:T10)
        n182 = call "RefreshTimerFGV.vi"("Command"=enum16{"Initialize", "Check Time", "Reset"}."Initialize", "Error In"=w408, "Ticker Multiplier"=10.0, "Refresh Period [s]"=30.0) -> ("Error Out"=w407:errorcluster)  [unwired: 5 in, 2 out]
      }
      frame "RequestData" {
        n183 = Unbundle By Name(w446) -> ("Queues.MHLClient"=w426:refnum<queue>)
        n184 = call "Request StatusFGV.vi"("Error In"=w424, "Command"=enum16{"Block", "Unblock", "Check Status"}."Block") -> ("Error Out"=w423:errorcluster)  [unwired: 8 in, 1 out]
        n185 = call "GenerateMethodURL.vi"("Method"=enum16{"Heartbeat", "GetSRs"}."GetSRs", "TestClientData"=w451) -> ("String"=w449:string)  [unwired: 9 in]
        n186 = call "GET.vi"("url"=w449, "error in (no error)"=w423, "timeout (10000)"=5000) -> ("body"=w448:string, "error out"=w419:errorcluster)  [unwired: 9 in, 2 out]
        n187 = Unflatten From XML(xml string=w448, type=T9 [] ("SRList"), error in (no error)=w419) -> (value=w445:T9, error out=w418:errorcluster)
        n188 = Unbundle By Name(w418) -> ("status"=w431:bool)
        n189 = call "ConnectionQuality.vi"("Error?"=w431) -> ("Last Update"=w428:timestamp, "Connection Quality"=w429:dbl)  [unwired: 9 in]
        n190 = call "Prepare Data for ParserSorter.vi"("Error In"=w418, "SRList"=w445) -> ("Error Out"=w442:errorcluster, "Prepared SR List"=w443:T5)  [unwired: 8 in]
        n191 = Bundle(cluster=T6 {"Connection Quality"=0.0, "Last Update"=timestamp(0 s since 1904-01-01)} ("Connection Status"), "Connection Quality"=w429, "Last Update"=w428) -> (w427:T6)
        n192 = Increment(x="AE Groups") -> (x+1=w414:i32[])
        n193 = Equal?(x="AE Level", y=enum16{"AE / ELP", "AE Intern"}."AE / ELP") -> (x = y?=w440:bool)
        n194 = call "Parse-Sort-Split.vi"("AE Groups"=w414, "Include High Priority?"=w440, "Error In"=w442, "SR List In"=w443) -> ("Error Out"=w437:errorcluster, "Unassigned SR List"=w434:T5, "Assigned SR List"=w438:T5)  [unwired: 5 in]
        n195 = call "EnqueueMessage(Single).vi"("Message Data"=w427, "Message"="UpdateConnectionStatus", "Message Queue"=w426) -> ("error out"=w420:errorcluster)  [unwired: 7 in, 1 out]
        n196 = call "EnqueueMessage(Single).vi"("error in (no error)"=w437, "Message Data"=w438, "Message"="UpdateAssignedSorted", "Message Queue"=w426) -> ("error out"=w436:errorcluster, "dup Message Queue"=w432:refnum<queue>)  [unwired: 6 in]
        n197 = flat-sequence {
          tunnel: w417 -> [w453]
          tunnel: [w453] -> w416
          frame #0 {
            n198 = call "RefreshTimerFGV.vi"("Command"=enum16{"Initialize", "Check Time", "Reset"}."Reset") -> ()  [unwired: 8 in, 3 out]
            n199 = call "Request StatusFGV.vi"("Command"=enum16{"Block", "Unblock", "Check Status"}."Unblock") -> ()  [unwired: 9 in, 2 out]
          }
        }
        n200 = call "EnqueueMessage(Single).vi"("error in (no error)"=w436, "Message Data"=w434, "Message"="UpdateUnassignedSorted", "Message Queue"=w432) -> ("error out"=w435:errorcluster)  [unwired: 6 in, 1 out]
        n201 = Merge Errors(w435, w420) -> (w417:errorcluster)
      }
      frame "Stop" {
      }
    }
    n202 = call "ErrorHandler.vi"("error in (no error)"=w357) -> ("error out"=w356:errorcluster)  [unwired: 10 in]
  }
  n203 = Merge Errors(w9, w8, w7, w6, w5, w2) -> (w10:errorcluster)
  n204 = call "DestroyCommunication.vi"("error in (no error)"=w10, "Message Queues"=w3) -> ("error out"=w1:errorcluster)  [unwired: 9 in]
  n205 = disable-structure shown="RUN_TIME_ENGINE==True" {
    disable-tunnel: w1 -> [_ _]
    frame condition #0 (active) {
    }
    frame condition #1 {
      # "Call Quit LabVIEW if running as a built application."
      n206 = Quit LabVIEW() -> ()  [unwired: 1 in]
    }
  }
